vi "Teleop.vi"(10 "Match Info":T1={"Autonomous Elapsed Seconds"=0.0, "TeleOp Elapsed Seconds"=0.0, "Disabled Elapsed Seconds"=0.0, "Visited Autonomous"=FALSE, "Visited TeleOp"=FALSE, "Visited Disabled"=FALSE, "Autonomous Settings"={"Autonomous Style"=enum."Independent", "VI Refnum"=refnum}}, 11 "Call Context":T2) -> ()   [LabVIEW 2012]
doc: "This VI is called for each TeleOp packet received from the DS where the robot is not disabled. It is often used to read from the joysticks and update I/O or to update setpoints for timed control loops. It should complete and return within 20 milliseconds or it may miss DS packets."
uses:
  <vilib>/Rock Robotics/WPI/DriverStation/WPI_DriverStationDerivedRobotMode.ctl
  <vilib>/Rock Robotics/WPI/DriverStation/WPI_DriverStationMatch Info.ctl
  <vilib>/Rock Robotics/WPI/Relay/WPI_RelayValue.ctl
  Robot Global Data.vi
  <vilib>/Rock Robotics/WPI/Joystick/WPI_JoystickGetSetRefNum.vi
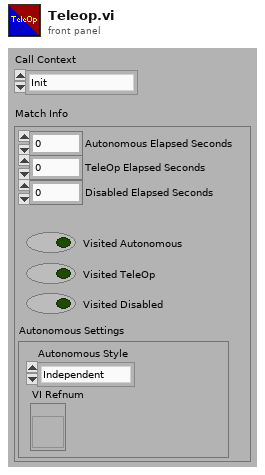
[diagram p1: front panel]
types:
  T1 = typedef "WPI_DriverStationMatch Info.ctl" = cluster{"Autonomous Elapsed Seconds":dbl, "TeleOp Elapsed Seconds":dbl, "Disabled Elapsed Seconds":dbl, "Visited Autonomous":bool, "Visited TeleOp":bool, "Visited Disabled":bool, "Autonomous Settings":cluster{"Autonomous Style":enum16{"Iterative", "Independent"}, "VI Refnum":refnum<vi>}}
  T2 = typedef "WPI_DriverStationDerivedRobotMode.ctl" = enum16{"Init", "Execute", "Stop"}
  T3 = typedef "WPI_RelayValue.ctl" = enum16{"Off", "On", "Forward", "Reverse"}
  T4 = typedef "WPI_JoystickDevRef.ctl" = cluster{"Device":T5}
  T5 = typedef "WPI_JoystickDeviceEnum.ctl" = enum16{"USB 1", "USB 2", "USB 3", "USB 4", "Kinect 1", "Kinect 2"}
  T6 = typedef "WPI_RelayDevRef.ctl" = cluster{"DevStatus":errorcluster, "Relay Channel":T7, "Digital Module":T8, "Relay Direction":T9}
  T7 = typedef "FPGA_DIORelayChannel.ctl" = enum8{"Relay 1", "Relay 2", "Relay 3", "Relay 4", "Relay 5", "Relay 6", "Relay 7", "Relay 8", "Invalid"}
  T8 = typedef "FPGA_TypedefDigitalModule.ctl" = enum16{"Digital Module 1", "Digital Module 2"}
  T9 = typedef "WPI_RelayDirection.ctl" = enum16{"Both directions", "Forward only", "Reverse only"}
  T10 = cluster{"axis 1 (x)":dbl, "axis 2 (y)":dbl, "axis 3 (throttle)":dbl, "axis 4":dbl, "axis 5":dbl, "axis 6":dbl}
  T11 = typedef "WPI_MotorControlDeviceRef.ctl" = cluster{"DeviceStatus":errorcluster, "Type":enum16{"PWM", "CAN"}, "PWM":cluster{"Digital Module":T8, "PWM Channel":T12, "DeadBand":T13}, "CAN":cluster{"Device Number":u8, "Control Mode":T14, "Semaphore":T15, "Max Vout":dbl}, "Invert":bool, "TransformRef":T16, "InvTransformRef":T16}
  T12 = typedef "FPGA_DIOPWMChannel.ctl" = enum8{"PWM 1", "PWM 2", "PWM 3", "PWM 4", "PWM 5", "PWM 6", "PWM 7", "PWM 8", "PWM 9", "PWM 10", "Invalid"}
  T13 = typedef "WPI_PWMDeadband.ctl" = cluster{"Name":string, "maxPositivePwm":i32, "minPositivePwm":i32, "centerPwm":i32, "maxNegativePwm":i32, "minNegativePwm":i32, "angularRange":u16}
  T14 = typedef "WPI_CANJaguar_ControlMode.ctl" = enum8{"Percent VBus", "Current", "Speed", "Position", "Voltage"}
  T15 = typedef "Semaphore RefNum" = refnum<k1>
  T16 = typedef "WPI_PWMTransform_ConPane.ctl" = refnum<vi>
  T17 = typedef "WPI_JoystickButtonState.ctl" = cluster{"Button 1":bool, "Button 2":bool, "Button 3":bool, "Button 4":bool, "Button 5":bool, "Button 6":bool, "Button 7":bool, "Button 8":bool, "Button 9":bool, "Button 10":bool, "Button 11":bool, "Button 12":bool}
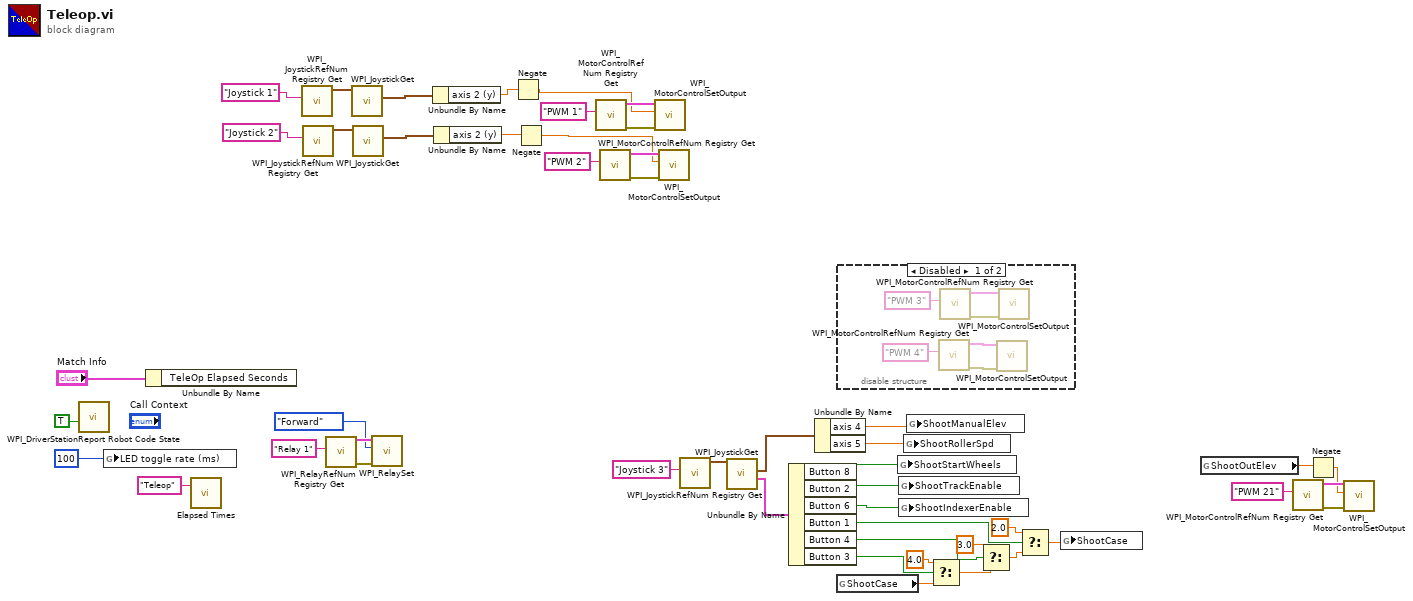
[diagram p0: block diagram]
diagram:
  n1 = call <vilib>:"WPI_DriverStationReport Robot Code State.vi"("TeleOp"=TRUE ("Autonomous")) -> ()  [unwired: 10 in, 1 out]
  n2 = global write "Robot Global Data.vi" "LED toggle rate (ms)"(u32 100 ("LED ms toggle rate")) -> ()
  n3 = Unbundle By Name("Match Info") -> ()  [unwired: 1 out]
  n4 = call "Elapsed Times.vi"("Call Name"="Teleop") -> ()  [unwired: 2 in, 1 out]
  n5 = call <vilib>:"WPI_JoystickRefNum Registry Get.vi"("refnum name"="Joystick 1") -> ("JoystickDevRef"=w15:T4)  [unwired: 1 in, 9 out]
  n6 = call <vilib>:"WPI_JoystickRefNum Registry Get.vi"("refnum name"="Joystick 2") -> ("JoystickDevRef"=w12:T4)  [unwired: 1 in, 9 out]
  n7 = call <vilib>:"WPI_RelayRefNum Registry Get.vi"("refnum name"="Relay 1") -> ("error out"=w43:errorcluster, "RelayDevRef"=w45:T6)  [unwired: 9 in]
  n8 = call <vilib>:"WPI_JoystickGet.vi"("JoystickDevRef"=w15) -> ("Axes"=w14:T10)  [unwired: 1 in, 5 out]
  n9 = call <vilib>:"WPI_JoystickGet.vi"("JoystickDevRef"=w12) -> ("Axes"=w13:T10)  [unwired: 1 in, 5 out]
  n10 = call <vilib>:"WPI_RelaySet.vi"("error in (no error)"=w43, "RelayValue"=WPI_RelayValue."Forward", "RelayDevRef"=w45) -> ()  [unwired: 7 in, 2 out]
  n11 = Unbundle By Name(w14) -> ("axis 2 (y)"=w2:dbl)
  n12 = Unbundle By Name(w13) -> ("axis 2 (y)"=w4:dbl)
  n13 = Negate(x=w2) -> (-x=w1:dbl)
  n14 = Negate(x=w4) -> (-x=w3:dbl)
  n15 = call <vilib>:"WPI_MotorControlRefNum Registry Get.vi"("refnum name"="PWM 1") -> ("error out"=w5:errorcluster, "MotorControlDevRef"=w6:T11)  [unwired: 9 in]
  n16 = call <vilib>:"WPI_MotorControlRefNum Registry Get.vi"("refnum name"="PWM 2") -> ("error out"=w10:errorcluster, "MotorControlDevRef"=w9:T11)  [unwired: 9 in]
  n17 = call <vilib>:"WPI_MotorControlSetOutput.vi"("error in (no error)"=w5, "Output"=w1, "MotorControlDevRef"=w6) -> ()  [unwired: 6 in, 3 out]
  n18 = call <vilib>:"WPI_MotorControlSetOutput.vi"("error in (no error)"=w10, "Output"=w3, "MotorControlDevRef"=w9) -> ()  [unwired: 6 in, 3 out]
  n19 = call <vilib>:"WPI_JoystickRefNum Registry Get.vi"("refnum name"="Joystick 3") -> ("JoystickDevRef"=w41:T4)  [unwired: 9 in, 1 out]
  n20 = call <vilib>:"WPI_JoystickGet.vi"("JoystickDevRef"=w41) -> ("Buttons"=w39:T17, "Axes"=w38:T10)  [unwired: 4 in, 1 out]
  n21 = Unbundle By Name(w39) -> ("Button 8"=w35:bool, "Button 2"=w36:bool, "Button 6"=w37:bool, "Button 1"=w32:bool, "Button 4"=w30:bool, "Button 3"=w29:bool)
  n22 = Unbundle By Name(w38) -> ("axis 4"=w34:dbl, "axis 5"=w33:dbl)
  n23 = global read "Robot Global Data.vi" "ShootCase"() -> (w24:dbl)
  n24 = disable-structure shown="Disabled" {
    frame Disabled {
      n25 = call <vilib>:"WPI_MotorControlRefNum Registry Get.vi"("refnum name"="PWM 4") -> ("error out"=w54:errorcluster, "MotorControlDevRef"=w53:T11)  [unwired: 9 in]
      n26 = call <vilib>:"WPI_MotorControlRefNum Registry Get.vi"("refnum name"="PWM 3") -> ("error out"=w49:errorcluster, "MotorControlDevRef"=w50:T11)  [unwired: 9 in]
      n27 = call <vilib>:"WPI_MotorControlSetOutput.vi"("error in (no error)"=w54, "MotorControlDevRef"=w53) -> ()  [unwired: 7 in, 3 out]
      n28 = call <vilib>:"WPI_MotorControlSetOutput.vi"("error in (no error)"=w49, "MotorControlDevRef"=w50) -> ()  [unwired: 7 in, 3 out]
    }
    frame Enabled {
    }
  }
  n29 = global write "Robot Global Data.vi" "ShootStartWheels"(w35) -> ()
  n30 = global write "Robot Global Data.vi" "ShootTrackEnable"(w36) -> ()
  n31 = global write "Robot Global Data.vi" "ShootIndexerEnable"(w37) -> ()
  n32 = global write "Robot Global Data.vi" "ShootRollerSpd"(w33) -> ()
  n33 = global write "Robot Global Data.vi" "ShootManualElev"(w34) -> ()
  n34 = Select(t=4.0, s=w29, f=w24) -> (s? t:f=w28:dbl)
  n35 = Select(t=3.0, s=w30, f=w28) -> (s? t:f=w26:dbl)
  n36 = Select(t=2.0, s=w32, f=w26) -> (s? t:f=w23:dbl)
  n37 = global write "Robot Global Data.vi" "ShootCase"(w23) -> ()
  n38 = global read "Robot Global Data.vi" "ShootOutElev"() -> (w19:dbl)
  n39 = call <vilib>:"WPI_MotorControlRefNum Registry Get.vi"("refnum name"="PWM 21") -> ("error out"=w22:errorcluster, "MotorControlDevRef"=w21:T11)  [unwired: 9 in]
  n40 = Negate(x=w19) -> (-x=w18:dbl)
  n41 = call <vilib>:"WPI_MotorControlSetOutput.vi"("error in (no error)"=w22, "Output"=w18, "MotorControlDevRef"=w21) -> ()  [unwired: 6 in, 3 out]
